vi "getNCv_short.vi"(4 "NC_var":T1 {"NC_attrarray"."nc_type" items=["NC_NAT", "NC_BYTE", "NC_CHAR", "NC_SHORT", "NC_INT", "NC_FLOAT", "NC_DOUBLE"]}, 5 "ErrorIn":errorcluster caption="错误输入", 6 "nelems":u64, 7 "start":u64[](array[numeric]), 8 "refnum":refnum<file>) -> (0 "ErrorOut":errorcluster caption="错误输出", 2 "value":i16[](array[numeric]), 3 "refnum out":refnum<file>)   [LabVIEW 2016]
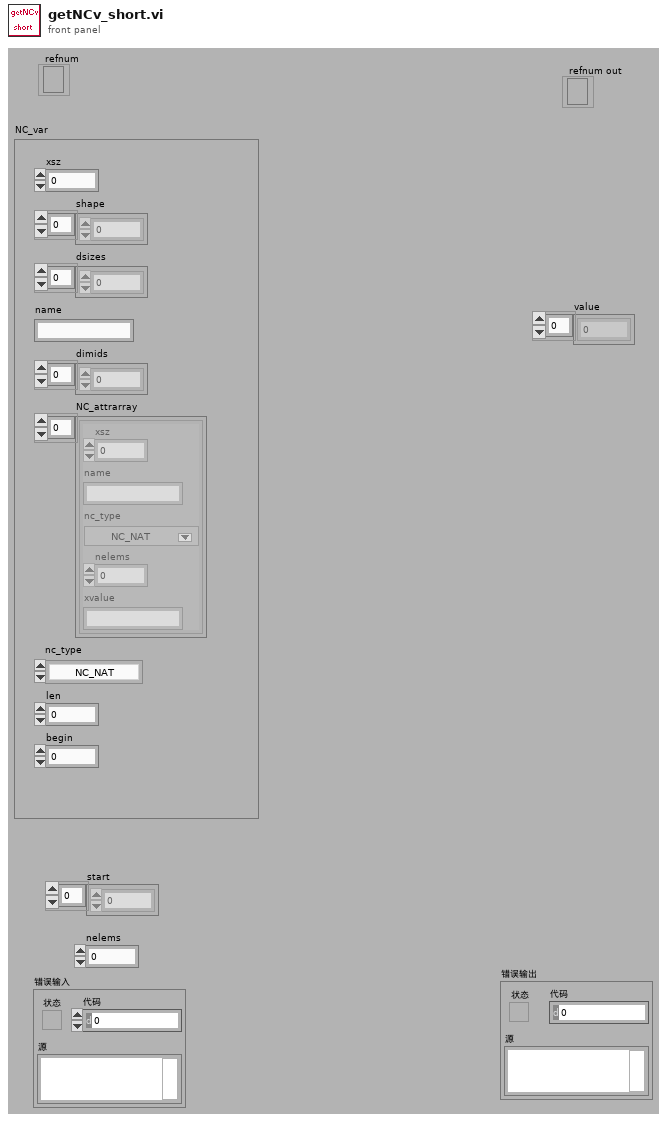
[diagram p1: front panel]
types:
  T1 = cluster{"xsz":u64, "shape":u64[], "dsizes":u64[], "name":string, "dimids":u64[], "NC_attrarray":cluster{"xsz":u64, "name":string, "nc_type":u16, "nelems":u64, "xvalue":string}[], "nc_type":enum16{"NC_NAT", "NC_BYTE", "NC_CHAR", "NC_SHORT", "NC_INT", "NC_FLOAT", "NC_DOUBLE"}, "len":u64, "begin":u64}
  T2 = enum16{"big-endian, network order", "native, host order", "little-endian"}
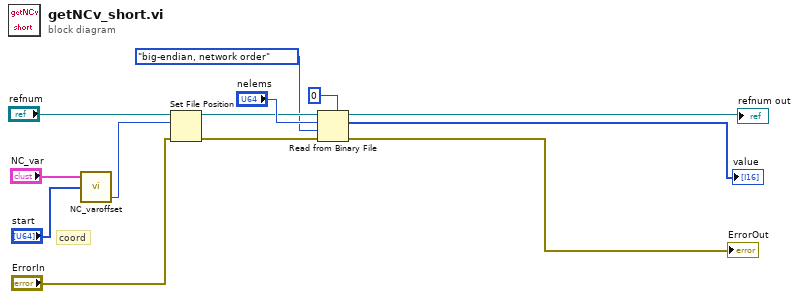
[diagram p0: block diagram]
diagram:
  # "coord"
  n1 = call "NC_varoffset.vi"("coord"="start", "NC_var"="NC_var") -> ("lcoord"=w1:u64)  [unwired: 3 out]
  n2 = Set File Position(offset (in bytes) (0)=w1, refnum="refnum", error in="ErrorIn") -> (refnum out=w9:refnum<file>, error out=w4:errorcluster)  [unwired: 1 out]
  n3 = Read from Binary File(5:i16 0, 8:w4, 9:T2."big-endian, network order" ("字节顺序(0:big-endian, network order)"), 10:"nelems", 11:w9) -> (0:→"ErrorOut":errorcluster, 2:→"value":i16[], 3:→"refnum out":refnum<file>)  [unwired: 2 out]
